vi "Set Sheets.vi"(8 "error in (no error)":errorcluster, 10 "Sheets":refnum<class "List.lvclass">[](array[class]), 11 "List_UI in":refnum<class "List_UI.lvclass">) -> (0 "error out":errorcluster, 3 "List_UI out":refnum<class "List_UI.lvclass">)   [LabVIEW 2015, in "List_UI.lvclass"]
uses:
  List_UI.lvclass
  resources/_list/List.lvclass
  List_UI.lvclass/List_UI.ctl
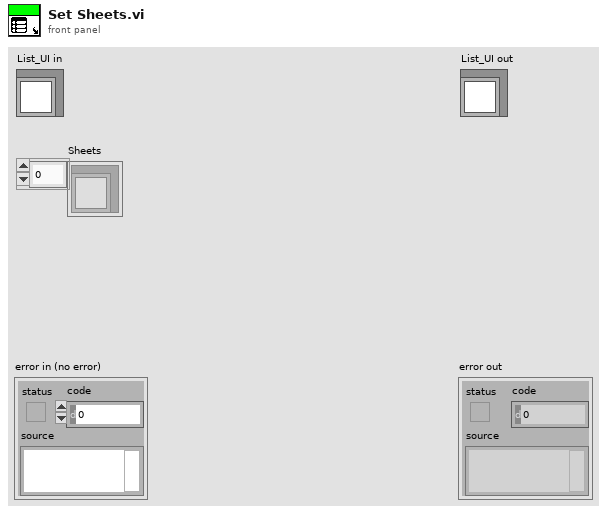
[diagram p1: front panel]
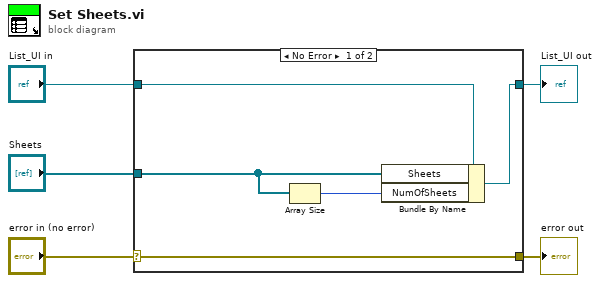
[diagram p0: block diagram]
diagram:
  n1 = case shown="No Error" "error in (no error)" {
    selector: "error in (no error)" -> [w10 w11]
    tunnel: [w10 w11] -> w4
    tunnel: [w8 w12] -> w2
    tunnel: "List_UI in" -> [w9 w12]
    tunnel: "Sheets" -> [w7 _]
    frame No Error {
      n2 = Array Size(array=w7) -> (size(s)=w6:i32)
      n3 = Bundle By Name(cluster=w9, "Sheets"=w7, "NumOfSheets"=w6) -> (w8:refnum<class "List_UI.lvclass">)
    }
    frame Error {
    }
  }
  "error out" <- w4
  "List_UI out" <- w2
